vi "Judge Siblings Symbols.vi"(8 "error in (no error)":errorcluster, 9 "Symbol":i32, 10 "Tag":string, 11 "TreeControl in":refnum<vi>) -> (0 "error out":errorcluster, 2 "The Same?":bool, 3 "TreeControl out":refnum<vi>)   [LabVIEW 2014, in "DSLV_Tree.lvlib"]
uses:
  DSLV_Tree.lvlib
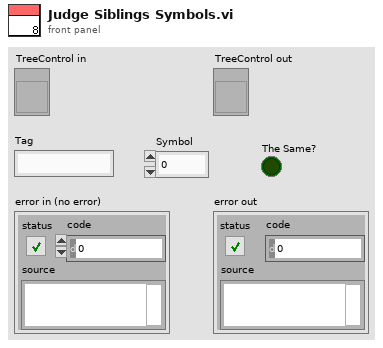
[diagram p1: front panel]
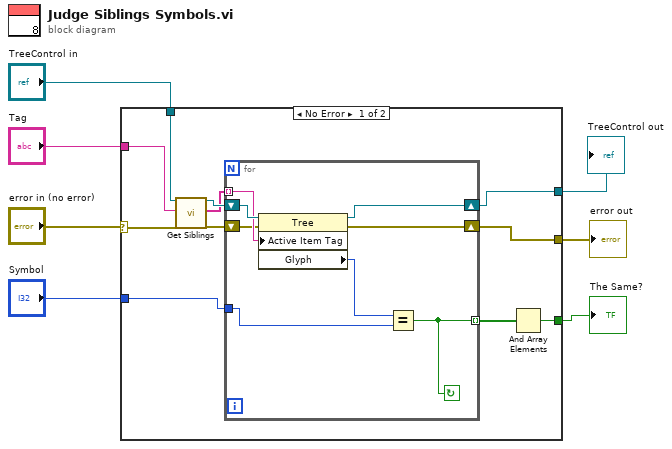
[diagram p0: block diagram]
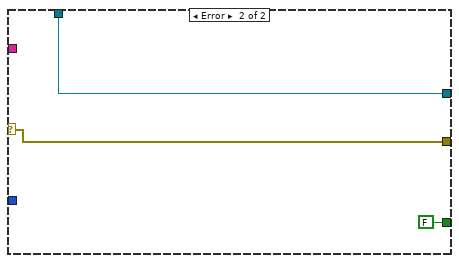
[diagram p2: hidden frame]
diagram:
  n1 = case shown="No Error" "error in (no error)" {
    selector: "error in (no error)" -> [w8 w28]
    tunnel: [w18 w28] -> w7
    tunnel: [w17 w29] -> w6
    tunnel: "Tag" -> [w13 _]
    tunnel: "TreeControl in" -> [w12 w29]
    tunnel: "Symbol" -> [w11 _]
    tunnel: [w9 FALSE] -> w2
    frame No Error {
      n2 = call "Get Siblings.vi"("Tree Reference In"=w12, "Input Tag (Current)"=w13, "error in (no error)"=w8) -> ("Tree Reference Out"=w16:refnum<vi>, "Sibling Tags"=w14:string[], "error out"=w15:errorcluster)  [unwired: 14 in]
      n3 = for {
        tunnel: w14 -> [w25] mode=indexing
        shift-right: [w22] -> w18
        shift-left: w15 -> [w24]
        shift-right: [w23] -> w17
        shift-left: w16 -> [w26]
        tunnel: w11 -> [w20]
        tunnel: [w19] -> w10 mode=indexing
        stop <- w19 continue-if-true
        n4 = property on="Property Node" class="Tree"(reference=w26, error in=w24, "Active Item Tag"=w25) -> (reference out=w23:refnum<vi>, error out=w22:errorcluster, "Glyph"=w21:i32)
        n5 = Equal?(x=w21, y=w20) -> (x = y?=w19:bool)
      }
      n6 = And Array Elements(Boolean array=w10) -> (logical AND=w9:bool)
    }
    frame Error {
    }
  }
  "error out" <- w7
  "TreeControl out" <- w6
  "The Same?" <- w2
